vi "SendSWtrigger.vi"(8 "error in":errorcluster, 11 "scope in":T1={"scope mode"=enum."Stopped", "ticker"=refnum, "5160 samples per trigger"=0, "FPGA ref"=refnum, "P2P params"={"instrument handle"="", "stream session"=refnum, "scale"={"offset"=0.0, "gain"=0.0, "reserved 1"=0.0, "reserved 2"=0.0}, "actual sample rate"=10000000.0, "Trigger"=enum."PFI 0", "SCOPE Resource"="Dev1", "input impedance"=0}, "data mode"=enum."Real IO", "5782 samples per record"=0, "Chart length"=0} {"P2P params"."input impedance" items=["1 mega ohm"=0, "50 ohms"=2]; "P2P params"."actual sample rate" format="%.2p"}) -> (0 "error out":errorcluster, 3 "scope out":T1={"scope mode"=enum."Stopped", "ticker"=refnum, "5160 samples per trigger"=0, "FPGA ref"=refnum, "P2P params"={"instrument handle"="", "stream session"=refnum, "scale"={"offset"=0.0, "gain"=0.0, "reserved 1"=0.0, "reserved 2"=0.0}, "actual sample rate"=10000000.0, "Trigger"=enum."PFI 0", "SCOPE Resource"="Dev1", "input impedance"=0}, "data mode"=enum."Real IO", "5782 samples per record"=0, "Chart length"=0} {"P2P params"."input impedance" items=["1 mega ohm"=0, "50 ohms"=2]; "P2P params"."actual sample rate" format="%.2p"})   [LabVIEW 2013]
uses:
  controls/scope_params.ctl
  Utilities/Ticker/Ticker.lvclass
  controls/ScopeMode.ctl
  Config/FPGAref.ctl
  P2P streaming/P2P params.ctl
  P2P streaming/trigger_source.ctl
  FPGA/DataMode.ctl
  <vilib>/rvi/interface/common/niFpgaWaitOnOcc.vi
  <vilib>/Utility/error.llb/Error Cluster From Error Code.vi
  <vilib>/rvi/errors/niLvFpgaAdjustHostInterfaceError.vi
  <vilib>/rvi/interface/nirviReadWriteControl/nirviReadWriteControl.xnode
  NiFpgaLv.dll
  <vilib>/rvi/interface/Simulation/niFpgaSimulationCallBeginRW.vi
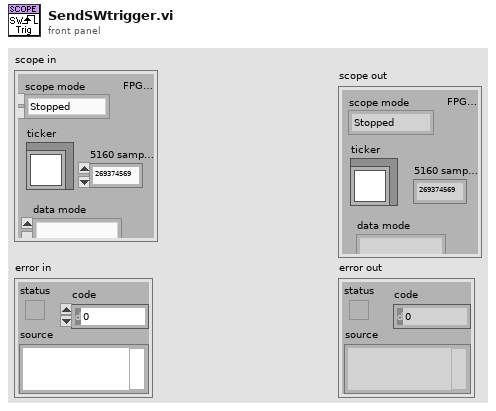
[diagram p1: front panel]
types:
  T1 = typedef "scope_params.ctl" = cluster{"scope mode":T2, "ticker":refnum<class "Ticker.lvclass">, "5160 samples per trigger":u32, "FPGA ref":T3, "P2P params":T4, "data mode":T6, "5782 samples per record":u32, "Chart length":i32}
  T2 = typedef "ScopeMode.ctl" = enum16{"Stopped", "Single", "Running", "Continuous"}
  T3 = typedef "FPGAref.ctl" = refnum<k20>
  T4 = typedef "P2P params.ctl" = cluster{"instrument handle":refnum<k15>, "stream session":refnum<k20>, "scale":cluster{"offset":dbl, "gain":dbl, "reserved 1":dbl, "reserved 2":dbl}, "actual sample rate":dbl, "Trigger":T5, "SCOPE Resource":refnum<k15>, "input impedance":u32}
  T5 = typedef "trigger_source.ctl" = enum16{"PFI 0", "PFI 1", "Software"}
  T6 = typedef "DataMode.ctl" = enum16{"Real IO", "Simulated"}
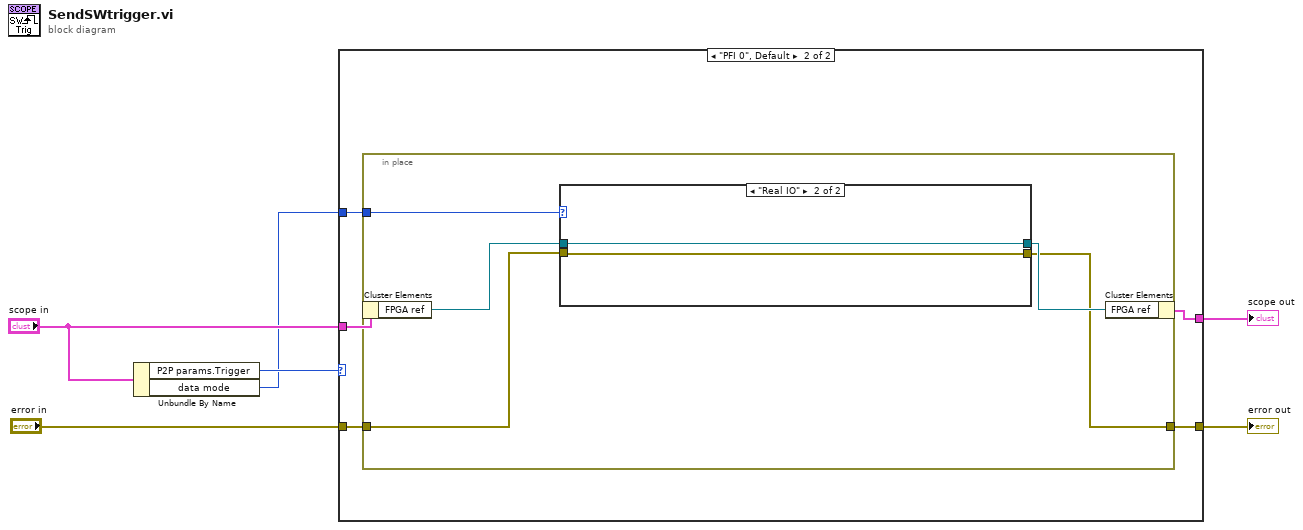
[diagram p0: block diagram]
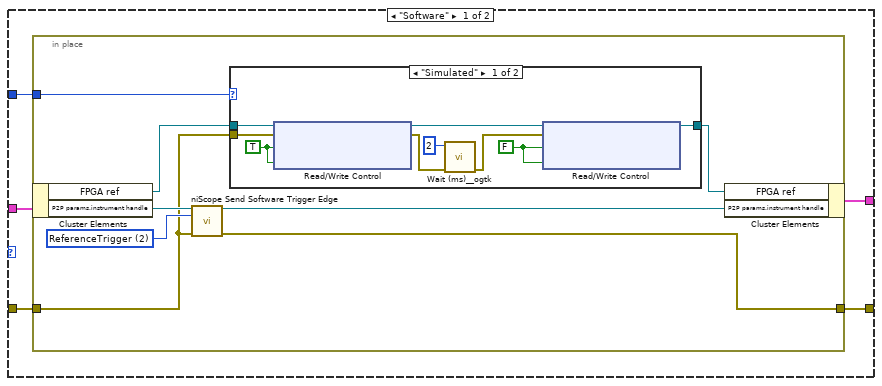
[diagram p2: hidden frame]
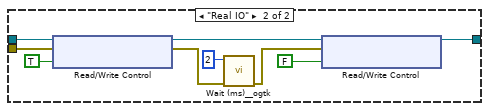
[diagram p3: hidden frame]
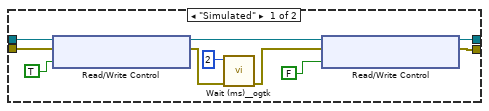
[diagram p4: hidden frame]
diagram:
  n1 = Unbundle By Name("scope in") -> ("P2P params.Trigger"=w6:T5, "data mode"=w3:T6)
  n2 = case shown="\"PFI 0\", Default" w6 {
    tunnel: "scope in" -> [w11 w42]
    tunnel: [w10 w41] -> w2
    tunnel: "error in" -> [w9 w40]
    tunnel: [w8 w39] -> w1
    tunnel: w3 -> [w7 w38]
    frame "Software" {
      n3 = in-place {
        in-place-border: w9 -> [w14]
        in-place-border: [w16] -> w8
        in-place-border: w7 -> [w13]
        w17 = u16 2 items=["StartTrigger", "ArmReferenceTrigger", "ReferenceTrigger", "AdvanceTrigger"] ("which trigger")
        n4 = in-place-cluster #1(w11) -> ("FPGA ref"=w15:T3, "P2P params.instrument handle"=w19:refnum<k15>)
        n5 = call <instrlib>:"niScope Send Software Trigger Edge.vi"("instrument handle"=w19, "which trigger"=w17, "error in"=w14) -> ("instrument handle out"=w18:refnum<k15>, "error out"=w16:errorcluster)  [unwired: 11 in]
        n6 = case shown="\"Simulated\"" w13 {
          tunnel: w15 -> [w25 w34]
          tunnel: [w24 w33] -> w12
          tunnel: w14 -> [w23 w32]
          frame "Simulated" {
            w20 = FALSE ("Trigger Acquisition")
            w21 = TRUE ("Trigger Acquisition")
            n7 = xnode "Read/Write Control"("FPGA VI Reference In"=w25, "error in"=w23, "Trigger Acquisition"=w21, "Trigger simulated data"=w21) -> ("FPGA VI Reference Out"=w28:T3, "error out"=w22:errorcluster)
            n8 = call <userlib>:"Wait (ms)__ogtk.vi"("error in (no error)"=w22, "milliseconds to wait"=u32 2) -> ("error out"=w27:errorcluster)  [unwired: 8 in, 1 out]
            n9 = xnode "Read/Write Control"("FPGA VI Reference In"=w28, "error in"=w27, "Trigger Acquisition"=w20, "Trigger simulated data"=w20) -> ("FPGA VI Reference Out"=w24:T3)  [unwired: 1 out]
          }
          frame "Real IO" {
            n10 = xnode "Read/Write Control"("FPGA VI Reference In"=w34, "error in"=w32, "Trigger Acquisition"=TRUE) -> ("FPGA VI Reference Out"=w37:T3, "error out"=w31:errorcluster)
            n11 = call <userlib>:"Wait (ms)__ogtk.vi"("error in (no error)"=w31, "milliseconds to wait"=u32 2) -> ("error out"=w36:errorcluster)  [unwired: 8 in, 1 out]
            n12 = xnode "Read/Write Control"("FPGA VI Reference In"=w37, "error in"=w36, "Trigger Acquisition"=FALSE) -> ("FPGA VI Reference Out"=w33:T3)  [unwired: 1 out]
          }
        }
        n13 = in-place-cluster #1("FPGA ref"=w12, "P2P params.instrument handle"=w18) -> (w10:T1)
      }
    }
    frame "PFI 0", Default {
      n14 = in-place {
        in-place-border: w40 -> [w46]
        in-place-border: [w43] -> w39
        in-place-border: w38 -> [w45]
        n15 = in-place-cluster #2(w42) -> ("FPGA ref"=w47:T3)
        n16 = case shown="\"Real IO\"" w45 {
          tunnel: w47 -> [w54 w59]
          tunnel: [w53 w59] -> w44
          tunnel: w46 -> [w52 w58]
          tunnel: [w48 w58] -> w43
          frame "Simulated" {
            n17 = xnode "Read/Write Control"("FPGA VI Reference In"=w54, "error in"=w52, "Trigger simulated data"=TRUE ("Trigger Acquisition")) -> ("FPGA VI Reference Out"=w57:T3, "error out"=w51:errorcluster)
            n18 = call <userlib>:"Wait (ms)__ogtk.vi"("error in (no error)"=w51, "milliseconds to wait"=u32 2) -> ("error out"=w56:errorcluster)  [unwired: 8 in, 1 out]
            n19 = xnode "Read/Write Control"("FPGA VI Reference In"=w57, "error in"=w56, "Trigger simulated data"=FALSE ("Trigger Acquisition")) -> ("FPGA VI Reference Out"=w53:T3, "error out"=w48:errorcluster)
          }
          frame "Real IO" {
          }
        }
        n20 = in-place-cluster #2("FPGA ref"=w44) -> (w41:T1)
      }
    }
  }
  "scope out" <- w2
  "error out" <- w1
